vi "Send Launch UI Message.vi"(8 "error in (no error)":errorcluster, 10 "User Interface.lvclass":refnum<class "UI.lvclass">, 11 "Message Enqueuer in":refnum<class "Message Enqueuer.lvclass">) -> (0 "error out":errorcluster, 3 "Message Enqueuer out":refnum<class "Message Enqueuer.lvclass">)   [LabVIEW 2016, in "Controller Actor.lvlib" / "Launch User Interface Msg.lvclass"]
uses:
  <userlib>/Common Components/Controller/Messages/Launch UI Message/Launch User Interface Msg.lvclass
  <userlib>/Common Components/User Interface/UI.lvclass
  <vilib>/ActorFramework/Message Enqueuer/Message Enqueuer.lvclass
  C:/Program Files (x86)/National Instruments/LabVIEW 2016/vi.lib/ActorFramework/Message/Message.lvclass
  <vilib>/ActorFramework/Message Enqueuer/Message Enqueuer.lvclass/Message Enqueuer.ctl
  <vilib>/ActorFramework/Message Priority Queue/Priority Enqueue.vi
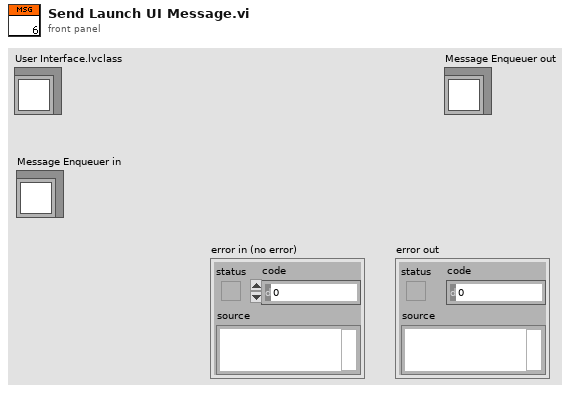
[diagram p1: front panel]
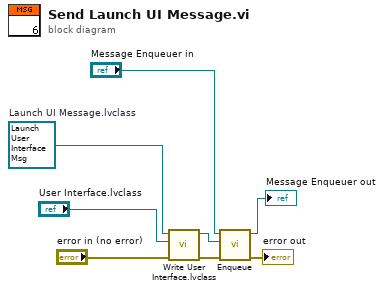
[diagram p0: block diagram]
diagram:
  w8 = refnum<class "Launch User Interface Msg.lvclass"> refnum  # Launch UI Message.lvclass
  n1 = call <userlib>:"Write User Interface.lvclass.vi"("error in (no error)"="error in (no error)", "User Interface.lvclass"="User Interface.lvclass", "Launch UI Message in"=w8) -> ("error out"=w2:errorcluster, "Launch UI Message out"=w6:refnum<class "Launch User Interface Msg.lvclass">)  [unwired: 7 in]
  n2 = call <vilib>:"Enqueue.vi"("error in (no error)"=w2, "Message"=w6, "Message Enqueuer in"="Message Enqueuer in") -> ("error out"=→"error out":errorcluster, "Message Enqueuer out"=→"Message Enqueuer out":refnum<class "Message Enqueuer.lvclass">)  [unwired: 7 in]
